vi "Test Noise Simulator.vi"() -> ()   [LabVIEW 2019, in "DAQmx.lvclass"]
uses:
  DAQmx.lvclass
  typedefs/DAQmx.Channel Map--Cluster.ctl
  typedefs/Simulation Mode--enum.ctl
  Instrument.DAQ/Typedefs/DAQ.Sampling.Sampling--Cluster.ctl
  Instrument.DAQ/Typedefs/DeviceInfo--Cluster.ctl
  DAQmx.lvclass/DAQmx.ctl
  Instrument.DAQ/Instrument.DAQ.lvclass
  <vilib>/measure/NI_MABase.lvlib
panel:
  out "Numeric":i32
  out "Noisy Signal Graph":waveform(dbl)[](graph)
  in  "stop":bool
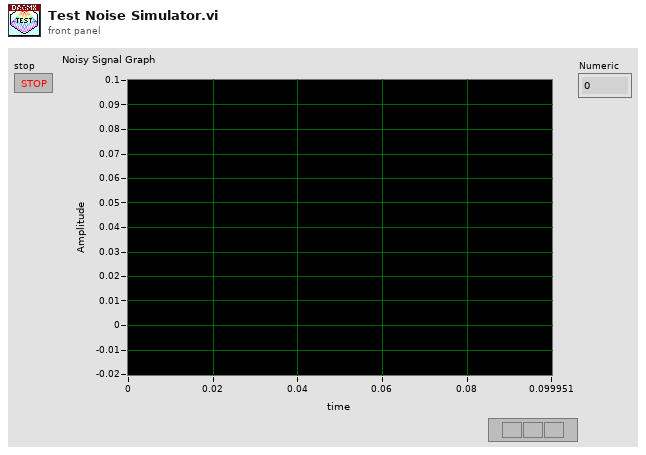
[diagram p1: front panel]
types:
  T1 = typedef "DAQmx.lvclass/DAQmx.Channel Map--Cluster.ctl" = cluster{"task":refnum<k21>, "Device":tag, "Offset":u32, "Count":u32, "DevIsSimulated":bool}
  T2 = typedef "DAQmx.lvclass/Simulation Mode--enum.ctl" = enum16{"AI = HW simulated", "AI = noise*AO", "AI = waveguide"}
  T3 = typedef "Instrument.Lockin.lvlib/Instrument.DAQ.lvclass/DAQ.Sampling.Sampling--Cluster.ctl" = cluster{"Fs":dbl, "#s":i32}
  T4 = typedef "Instrument.Lockin.lvlib/Instrument.DAQ.lvclass/DeviceInfo--Cluster.ctl" = cluster{"DeviceName":string, "DevIsSimulated":bool, "DeviceSerialNumber":string, "ProductType":string, "ProductCategory":i32, "ProductNumber":u32, "ChassisNumber":u32, "SlotNumber":u32, "ChassisName":string, "ChassisSerialNumber":string, "DevTemp":dbl, "SelfCal.LastDate/Time":string, "SelfCal.LastTemp":dbl, "calibration due?":bool}
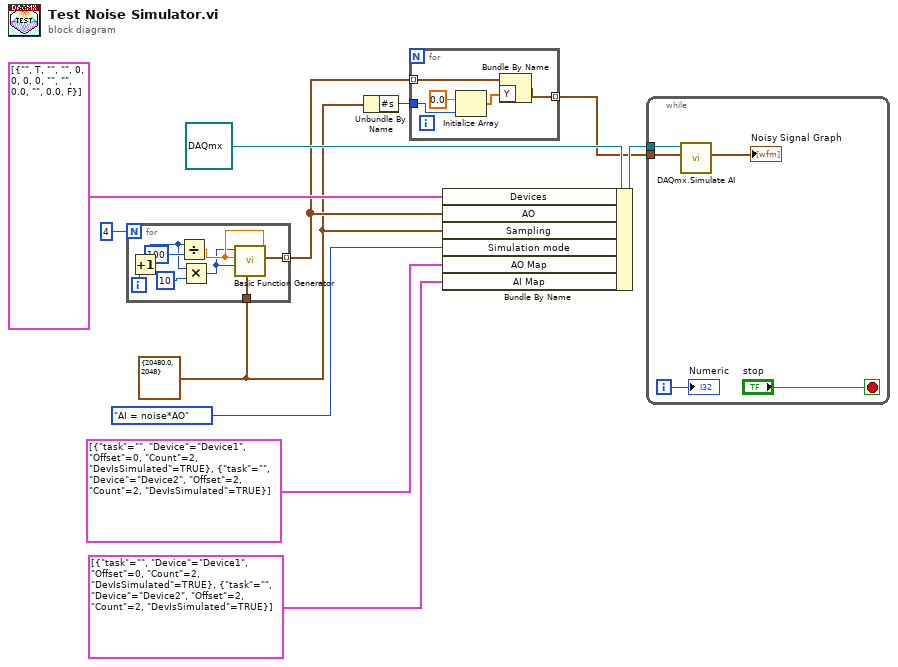
[diagram p0: block diagram]
diagram:
  w2 = T3 {"Fs"=20480.0, "#s"=2048} ("Configuration.DAQ.Sampling.Sampling")
  n1 = for {
    N: 4 -> [_]
    tunnel: w2 -> [w19]
    tunnel: [w18] -> w4 mode=indexing
    i -> [w17]
    n2 = Increment(x=w17) -> (x+1=w14:i32)
    n3 = Divide(x=w14, y=100) -> (x/y=w13:dbl)
    n4 = Multiply(x=w14, y=10) -> (x*y=w12:i32)
    n5 = call <vilib>:"Basic Function Generator.vi"("offset"=w13, "sampling info"=w19, "phase"=w12, "amplitude"=w13, "frequency"=w12) -> ("signal out"=w18:waveform(dbl))  [unwired: 4 in, 2 out]
  }
  n6 = Unbundle By Name(w2) -> ("#s"=w1:i32)
  n7 = for {
    tunnel: w4 -> [w23] mode=indexing
    tunnel: [w24] -> w3 mode=indexing
    tunnel: w1 -> [w20]
    n8 = Initialize Array(0.0 ("element"), w20) -> (w21:dbl[])
    n9 = Bundle By Name(cluster=w23, "Y"=w21) -> (w24:waveform(dbl))
  }
  n10 = Bundle By Name(cluster=refnum<class "DAQmx.lvclass"> refnum ("DAQmx.lvclass"), "Devices"=T4[] [{"DeviceName"="", "DevIsSimulated"=TRUE, "DeviceSerialNumber"="", "ProductType"="", "ProductCategory"=0, "ProductNumber"=0, "ChassisNumber"=0, "SlotNumber"=0, "ChassisName"="", "ChassisSerialNumber"="", "DevTemp"=0.0, "SelfCal.LastDate/Time"="", "SelfCal.LastTemp"=0.0, "calibration due?"=FALSE}] ("Configuration.DAQ.Devices"), "AO"=w4, "Sampling"=w2, "Simulation mode"=Simulation_Mode--enum."AI = noise*AO" ("Configuration.DAQ.Simulation mode"), "AO Map"=T1[] [{"task"="", "Device"="Device1", "Offset"=0, "Count"=2, "DevIsSimulated"=TRUE}, {"task"="", "Device"="Device2", "Offset"=2, "Count"=2, "DevIsSimulated"=TRUE}], "AI Map"=T1[] [{"task"="", "Device"="Device1", "Offset"=0, "Count"=2, "DevIsSimulated"=TRUE}, {"task"="", "Device"="Device2", "Offset"=2, "Count"=2, "DevIsSimulated"=TRUE}]) -> (w11:refnum<class "DAQmx.lvclass">)
  n11 = while {
    tunnel: w11 -> [w29]
    tunnel: w3 -> [w25]
    i -> [w26]
    stop <- "stop" stop-if-true
    n12 = call "DAQmx.Simulate AI.vi"("AIwfm in"=w25, "DAQmx in"=w29) -> ("AIwfm out"=→"Noisy Signal Graph":waveform(dbl)[])  [unwired: 6 in, 3 out]
    "Numeric" <- w26
  }
